vi "Initialize Settings.vi"(11 "error in (no error)":errorcluster) -> (4 "Name":string, 6 "Plugins Folder 2":path, 8 "Data Logging Folder 2":path, 10 "bool":bool, 15 "error out":errorcluster)   [LabVIEW 2013, in "Manager.lvlib" / "Manager.lvclass"]
uses:
  Manager.lvclass
panel:
  in  "Plugins Folder":path
  in  "Data Logging Folder":path
  in  "Cancel Button":bool
  in  "Control System Name":string
  in  "Button":bool
  # "Enter System Parameters"
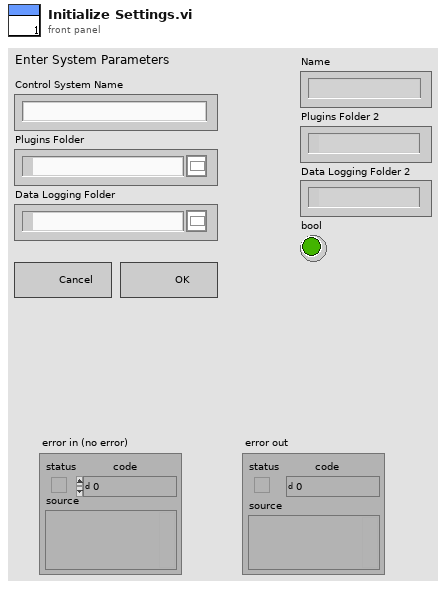
[diagram p1: front panel]
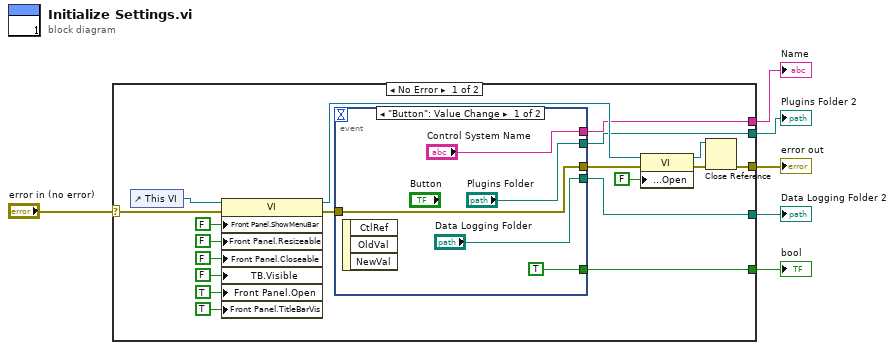
[diagram p0: block diagram]
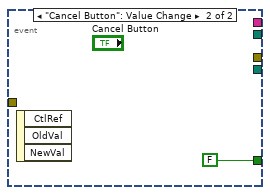
[diagram p2: hidden frame]
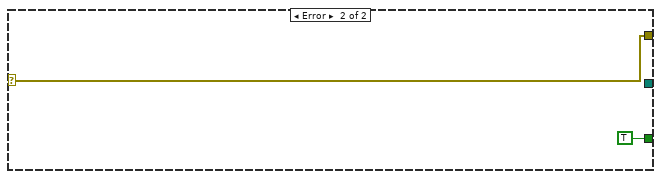
[diagram p3: hidden frame]
diagram:
  n1 = case shown="No Error" "error in (no error)" {
    selector: "error in (no error)" -> [w18 w33]
    tunnel: [w13 w33] -> w5
    tunnel: [w10 TRUE ("Front Panel Window:Open")] -> w4
    tunnel: [w9 _] -> w3
    tunnel: [w8 _] -> w1
    tunnel: [w7 _] -> w2
    frame No Error {
      n2 = control-ref of="This VI"() -> (w25:refnum<vi>)
      n3 = property class="VI"(reference=w25, error in=w18, "Front Panel.ShowMenuBar"=FALSE ("Front Panel Window:Show Menu Bar"), "Front Panel.Resizeable"=FALSE ("Front Panel Window:Resizable"), "Front Panel.Closeable"=FALSE ("Front Panel Window:Closeable"), "TB.Visible"=FALSE ("Tool Bar:Visible"), "Front Panel.Open"=TRUE ("Front Panel Window:Open"), "Front Panel.TitleBarVis"=TRUE ("Front Panel Window:Title Bar Visible")) -> (reference out=w12:refnum<vi>, error out=w17:errorcluster)
      n4 = event shown="[0] \"Button\": Value Change" {
        selector: _ -> [_ _]
        dyn-events: _ -> [_ _]
        timeout: _ -> [_ _]
        tunnel: w17 -> [w30 _]
        tunnel: [w30 _] -> w11
        tunnel: [TRUE ("Front Panel Window:Open") FALSE ("Front Panel Window:Open")] -> w10
        tunnel: ["Control System Name" _] -> w9
        tunnel: ["Data Logging Folder" _] -> w8
        tunnel: ["Plugins Folder" _] -> w7
        event "Button": Value Change {
          n5 = event-data() -> ()  [unwired: 1 in, 3 out]
        }
        event "Cancel Button": Value Change {
          n6 = event-data() -> ()  [unwired: 1 in, 3 out]
        }
      }
      n7 = property class="VI"(reference=w12, error in=w11, "Front Panel.Open"=FALSE ("Front Panel Window:Open")) -> (reference out=w16:refnum<vi>, error out=w15:errorcluster)
      n8 = Close Reference(reference=w16, error in (no error)=w15) -> (error out=w13:errorcluster)
    }
    frame Error {
    }
  }
  "error out" <- w5
  "bool" <- w4
  "Name" <- w3
  "Plugins Folder 2" <- w2
  "Data Logging Folder 2" <- w1
